vi "startSweepAndWait.vi"(8 "error in (no error)":errorcluster, 10 "Configure Sweep":T1 {"Sweep IV Step (V)" format="%#_6p"; "Sweep End (V)" format="%#_6p"; "Sweep Start (V)" format="%#_6p"; "Sweep Lockin Time (s)" format="%#_6p"}, 11 "Instrument.Lockin in":refnum<class "Instrument.Lockin.lvclass">) -> (0 "error out":errorcluster, 2 "SweepResults":T2, 3 "Instrument.Lockin out":refnum<class "Instrument.Lockin.lvclass">)   [LabVIEW 2016, in "Instrument.Lockin.lvclass"]
uses:
  Instrument.Lockin.lvclass
  Lockin.DAQ/Typedefs/SweepResults--Cluster.ctl
  Lockin.DAQ/Typedefs/Sweep Configuration--Cluster.ctl
  Lockin.DAQ/Typedefs/State-enum.ctl
  Lockin.DAQ/Lockin.DAQ.lvclass
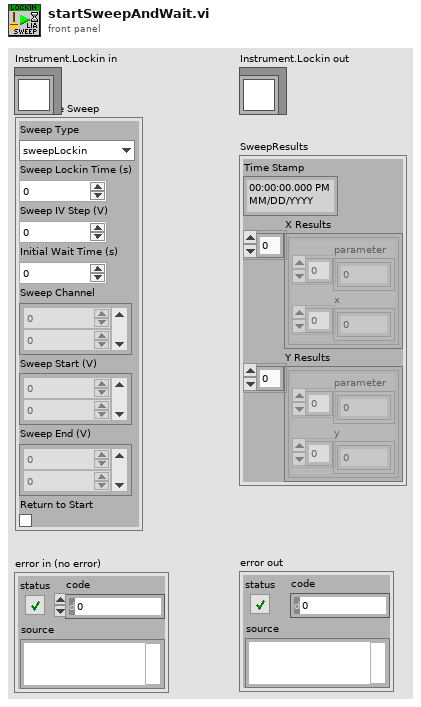
[diagram p1: front panel]
types:
  T1 = typedef "Lockin.DAQ.lvclass/Sweep Configuration--Cluster.ctl" = cluster{"Sweep Type":enum16{"sweepLockin", "sweepIV"}, "Sweep Lockin Time (s)":dbl, "Sweep IV Step (V)":dbl, "Initial Wait Time (s)":dbl, "Sweep Channel":i32[], "Sweep Start (V)":dbl[], "Sweep End (V)":dbl[], "Return to Start":bool}
  T2 = typedef "Lockin.DAQ.lvclass/SweepResults--Cluster.ctl" = cluster{"Time Stamp":timestamp, "X Results":cluster{"parameter":dbl[], "x":dbl[]}[], "Y Results":cluster{"parameter":dbl[], "y":dbl[]}[]}
  T3 = typedef "Lockin.DAQ.lvclass/State-enum.ctl" = enum16{"idle", "created", "started", "stopped", "sweeping"}
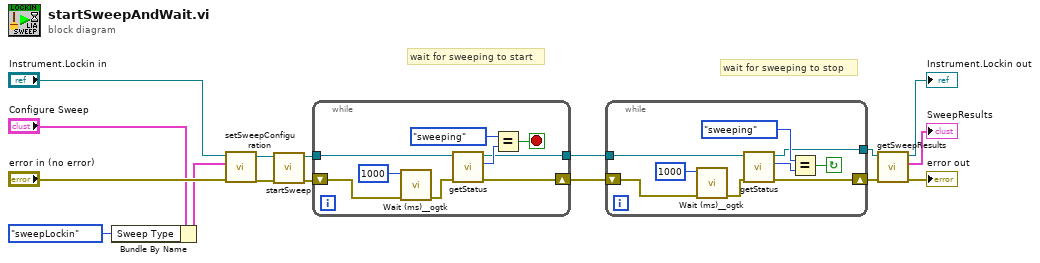
[diagram p0: block diagram]
diagram:
  # "wait for sweeping to stop"
  # "wait for sweeping to start"
  n1 = Bundle By Name(cluster="Configure Sweep", "Sweep Type"=enum16{"sweepLockin", "sweepIV"}."sweepLockin") -> (w1:T1)
  n2 = call "setSweepConfiguration.vi"("error in (no error)"="error in (no error)", "Configure Sweep"=w1, "Instrument.Lockin in"="Instrument.Lockin in") -> ("error out"=w7:errorcluster, "Instrument.Lockin out"=w8:refnum<class "Instrument.Lockin.lvclass">)  [unwired: 7 in]
  n3 = call "startSweep.vi"("error in (no error)"=w7, "Instrument.Lockin in"=w8) -> ("error out"=w5:errorcluster, "Instrument.Lockin out"=w6:refnum<class "Instrument.Lockin.lvclass">)  [unwired: 8 in]
  n4 = while {
    shift-right: [w25] -> w10
    shift-left: w5 -> [w17]
    tunnel: w6 -> [w21]
    tunnel: [w20] -> w9
    stop <- w22 stop-if-true
    n5 = call <userlib>:"Wait (ms)__ogtk.vi"("error in (no error)"=w17, "milliseconds to wait"=u32 1000) -> ("error out"=w19:errorcluster)  [unwired: 8 in, 1 out]
    n6 = call "getStatus.vi"("error in (no error)"=w19, "Instrument.Lockin"=w21) -> ("error out"=w25:errorcluster, "Status"=w24:T3, "Instrument.Lockin"=w20:refnum<class "Instrument.Lockin.lvclass">)  [unwired: 7 in]
    n7 = Equal?(x=State-enum."sweeping", y=w24) -> (x = y?=w22:bool)
  }
  n8 = while {
    shift-right: [w34] -> w13
    shift-left: w10 -> [w26]
    tunnel: w9 -> [w30]
    tunnel: [w29] -> w15
    stop <- w31 continue-if-true
    n9 = call <userlib>:"Wait (ms)__ogtk.vi"("error in (no error)"=w26, "milliseconds to wait"=u32 1000) -> ("error out"=w28:errorcluster)  [unwired: 8 in, 1 out]
    n10 = call "getStatus.vi"("error in (no error)"=w28, "Instrument.Lockin"=w30) -> ("error out"=w34:errorcluster, "Status"=w33:T3, "Instrument.Lockin"=w29:refnum<class "Instrument.Lockin.lvclass">)  [unwired: 7 in]
    n11 = Equal?(x=State-enum."sweeping", y=w33) -> (x = y?=w31:bool)
  }
  n12 = call "getSweepResults.vi"("error in (no error)"=w13, "Instrument.Lockin in"=w15) -> ("error out"=→"error out":errorcluster, "SweepResults"=→"SweepResults":T2, "Instrument.Lockin out"=→"Instrument.Lockin out":refnum<class "Instrument.Lockin.lvclass">)  [unwired: 7 in]
